vi "MotionProfileGeneratorVelocity.vi"(1 "Maximum Travel Speed (rps)":dbl, 2 "FL2":dbl, 3 "filter2sum":dbl, 4 "Filter1Sum":dbl) -> (0 "Velocity":dbl)   [LabVIEW 2017]
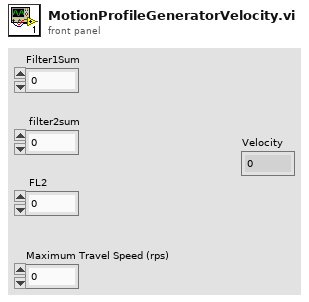
[diagram p1: front panel]
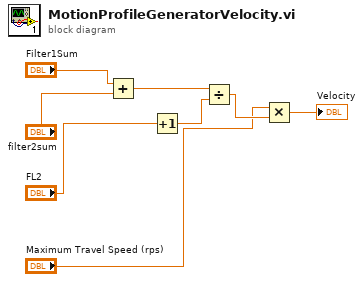
[diagram p0: block diagram]
diagram:
  n1 = Add(x="Filter1Sum", y="filter2sum") -> (x+y=w8:dbl)
  n2 = Increment(x="FL2") -> (x+1=w7:dbl)
  n3 = Divide(x=w8, y=w7) -> (x/y=w6:dbl)
  n4 = Multiply(x="Maximum Travel Speed (rps)", y=w6) -> (x*y=→"Velocity":dbl)
